vi "bubble_sort.vi"() -> ()   [LabVIEW 2021]
panel:
  out "sorted":dbl[](array[numeric])
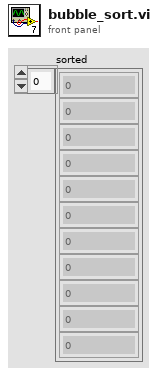
[diagram p1: front panel]
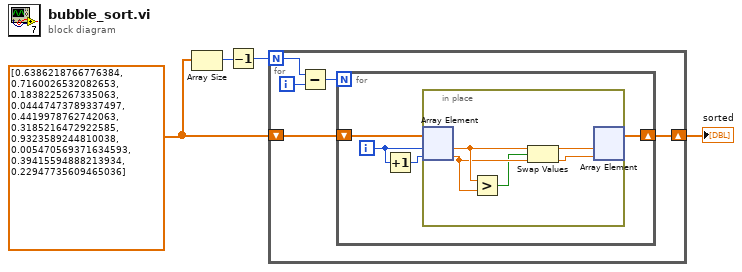
[diagram p0: block diagram]
diagram:
  w1 = dbl[] [0.6386218766776384, 0.7160026532082653, 0.1838225267335063, 0.04447473789337497, 0.4419978762742063, 0.3185216472922585, 0.9323589244810038, 0.005470569371634593, 0.39415594888213934, 0.22947735609465036] ("unsorted")
  n1 = Array Size(array=w1) -> (size(s)=w2:i32)
  n2 = Decrement(x=w2) -> (x-1=w4:i32)
  n3 = for {
    N: w4 -> [w9]
    shift-right: [w5] -> w3
    shift-left: w1 -> [w6]
    i -> [w7]
    n4 = Subtract(x=w9, y=w7) -> (x-y=w8:i32)
    n5 = for {
      N: w8 -> [_]
      shift-right: [w10] -> w5
      shift-left: w6 -> [w13]
      i -> [w12]
      n6 = Increment(x=w12) -> (x+1=w11:i32)
      n7 = in-place {
        n8 = in-place-array #1(w13, w12, w11) -> (w18:dbl, w17:dbl)
        n9 = Greater?(x=w18, y=w17) -> (0:w16:bool)
        n10 = Swap Values(12:w18, 13:w16, 14:w17) -> (1:w15:dbl, 3:w14:dbl)
        n11 = in-place-array #1(w15, w14) -> (w10:dbl[])  [unwired: 2 out]
      }
    }
  }
  "sorted" <- w3
